vi "serialize-xml.vi"() -> ()   [LabVIEW 2013]
uses:
  classes/MsgSerializer.XML/MsgSerializer.XML.lvclass
  classes/MsgSerializer.XML/format -- enum.ctl
  classes/MsgSerializer.XML/MsgSerializer.XML.lvclass/MsgSerializer.XML.ctl
panel:
  out "Serialized Test Case":string
  out "Serialized Test Suite":string
  out "Serialized Cluster":string
  out "Serialized Variant Attributes":string
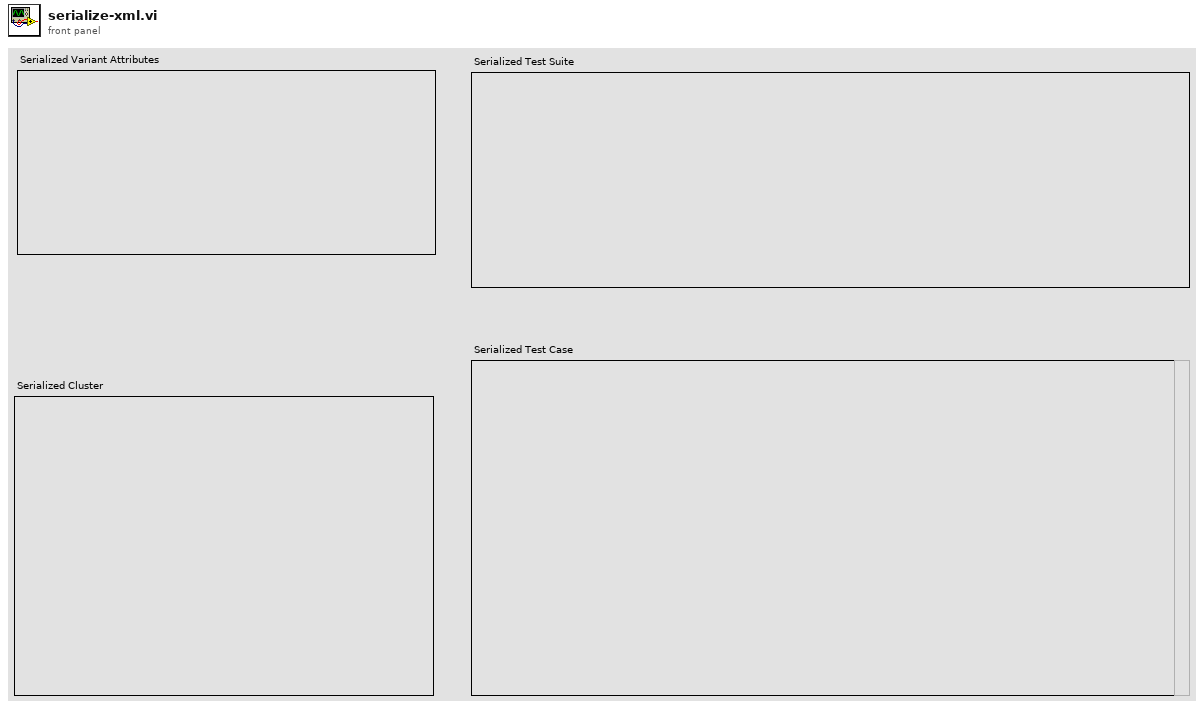
[diagram p1: front panel]
types:
  T1 = typedef "Caraya.lvlib/MsgSerializer.XML.lvclass/format -- enum.ctl" = enum16{"value", "tag", "property"}
  T2 = cluster{"classname":string, "name":string, "time":dbl, "skipped":bool, "failure":bool, "failure message":string, "failure description":string, "properties":variant, "measurements":variant, "limits":variant}[]
  T3 = cluster{"name":string, "errors":u32, "skipped":u32, "tests":u32, "failures":u32, "time":dbl, "timestamp":timestamp, "Call Chain":string[], "properties":variant}
  T4 = cluster{"status":bool, "code":i32, "inner":cluster{"status":bool, "code":i32, "timestamp":timestamp, "properties":variant}, "class":refnum<class "MsgSerializer.XML.lvclass">}
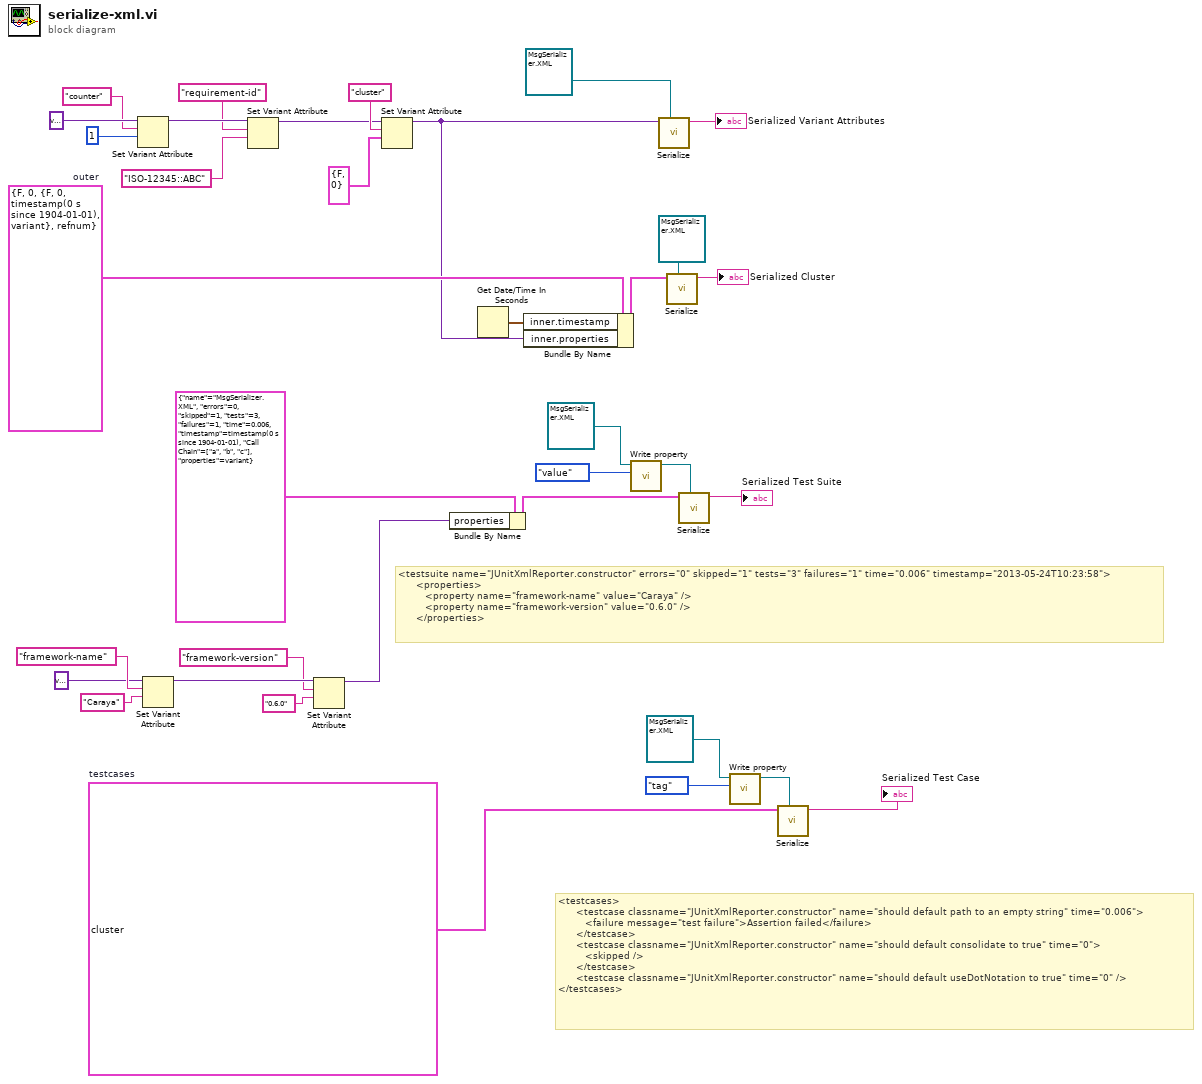
[diagram p0: block diagram]
diagram:
  w3 = T2 [{"classname"="MsgSerializer.XML", "name"="should default path to an empty string", "time"=0.006, "skipped"=FALSE, "failure"=TRUE, "failure message"="test failure", "failure description"="", "properties"=variant, "measurements"=variant, "limits"=variant}, {"classname"="MsgSerializer.XML", "name"="should default useDotNotation to true", "time"=0.0, "skipped"=FALSE, "failure"=FALSE, "failure message"="", "failure description"="", "properties"=variant, "measurements"=variant, "limits"=variant}, {"classname"="MsgSerializer.XML", "name"="should default consolidate to true", "time"=0.0, "skipped"=FALSE, "failure"=FALSE, "failure message"="", "failure description"="", "properties"=variant, "measurements"=variant, "limits"=variant}]  # testcases
  w22 = T4 {"status"=FALSE, "code"=0, "inner"={"status"=FALSE, "code"=0, "timestamp"=timestamp(0 s since 1904-01-01), "properties"=variant}, "class"=refnum}  # outer
  # "<testcases>\n      <testcase classname=\"JUnitXmlReporter.constructor\" name=\"should default path to an empty string\" time=\"0.006\">\n         <failure message=\"test failure\">Assertion failed</failure>\n      </testcase>\n      <testcase classname=\"JUnitXmlReporter.constructor\" name=\"should default consolidate to true\" time=\"0\">\n         <skipped />\n      </testcase>\n      <testcase classname=\"JUnitXmlReporter.constructor\" name=\"should default useDotNotation to true\" time=\"0\" />\n</testcases>"
  # "<testsuite name=\"JUnitXmlReporter.constructor\" errors=\"0\" skipped=\"1\" tests=\"3\" failures=\"1\" time=\"0.006\" timestamp=\"2013-05-24T10:23:58\">\n      <properties>\n         <property name=\"framework-name\" value=\"Caraya\" />\n         <property name=\"framework-version\" value=\"0.6.0\" />\n      </properties>"
  n1 = Set Variant Attribute(Variant=variant ("variant"), name="counter", value=1) -> (Variant out=w33:variant)  [unwired: 1 in, 2 out]
  n2 = Set Variant Attribute(Variant=variant ("variant"), name="framework-name", value="Caraya" ("name")) -> (Variant out=w14:variant)  [unwired: 1 in, 2 out]
  n3 = Set Variant Attribute(Variant=w33, name="requirement-id", value="ISO-12345::ABC" ("name")) -> (Variant out=w20:variant)  [unwired: 1 in, 2 out]
  n4 = Set Variant Attribute(Variant=w14, name="framework-version", value="0.6.0" ("name")) -> (Variant out=w12:variant)  [unwired: 1 in, 2 out]
  n5 = Set Variant Attribute(Variant=w20, name="cluster", value=cluster{"status":bool, "code":i32} {"status"=FALSE, "code"=0} ("error constant")) -> (Variant out=w1:variant)  [unwired: 1 in, 2 out]
  n6 = Bundle By Name(cluster=T3 {"name"="MsgSerializer.XML", "errors"=0, "skipped"=1, "tests"=3, "failures"=1, "time"=0.006, "timestamp"=timestamp(0 s since 1904-01-01), "Call Chain"=["a", "b", "c"], "properties"=variant} ("testsuite"), "properties"=w12) -> (w10:T3)
  n7 = Get Date/Time In Seconds() -> (seconds since 1Jan1904=w23:timestamp)
  n8 = Bundle By Name(cluster=w22, "inner.timestamp"=w23, "inner.properties"=w1) -> (w21:T4)
  n9 = call "Write property.vi"("format"=format_--_enum."value", "MsgSerializer.XMLProperty in"=refnum<class "MsgSerializer.XML.lvclass"> refnum ("Caraya.lvlib:MsgSerializer.XMLProperty.lvclass")) -> ("MsgSerializer.XMLProperty out"=w7:refnum<class "MsgSerializer.XML.lvclass">)  [unwired: 9 in]
  n10 = call-dynamic "Serialize.vi"("MsgSerializer"=refnum<class "MsgSerializer.XML.lvclass"> refnum ("Caraya.lvlib:MsgSerializer.XMLProperty.lvclass"), "Value"=w1) -> ("Serialized Message"=→"Serialized Variant Attributes":string)  [unwired: 8 in, 1 out]
  n11 = call-dynamic "Serialize.vi"("MsgSerializer"=refnum<class "MsgSerializer.XML.lvclass"> refnum ("Caraya.lvlib:MsgSerializer.XMLProperty.lvclass"), "Value"=w21) -> ("Serialized Message"=→"Serialized Cluster":string)  [unwired: 8 in, 1 out]
  n12 = call-dynamic "Serialize.vi"("MsgSerializer"=w7, "Value"=w10) -> ("Serialized Message"=→"Serialized Test Suite":string)  [unwired: 8 in, 1 out]
  n13 = call "Write property.vi"("format"=format_--_enum."tag", "MsgSerializer.XMLProperty in"=refnum<class "MsgSerializer.XML.lvclass"> refnum ("Caraya.lvlib:MsgSerializer.XMLProperty.lvclass")) -> ("MsgSerializer.XMLProperty out"=w6:refnum<class "MsgSerializer.XML.lvclass">)  [unwired: 9 in]
  n14 = call-dynamic "Serialize.vi"("MsgSerializer"=w6, "Value"=w3) -> ("Serialized Message"=→"Serialized Test Case":string)  [unwired: 8 in, 1 out]
